vi "Diconnect.vi"(4 "error in (no error)":errorcluster, 7 "VISA resource name":refnum<visa-resource-name>) -> ()   [LabVIEW 2015]
doc: "Funcitonally the opposite of the connect block. Use this to end communication with the ESP301. This is necessary but I am not sure why."
uses:
  <userlib>/Newport ESP301/Newport ESP301.lvlib
panel:
  # "This does the opposite of the Connect Block. \nNeeds to be run at the end of any program\nwhere  you have been communicating with \nthe ESP301 box."
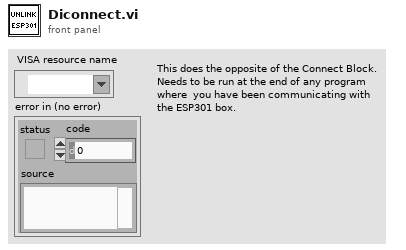
[diagram p1: front panel]
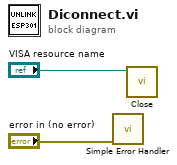
[diagram p0: block diagram]
diagram:
  n1 = call <vilib>:"Simple Error Handler.vi"("error in (no error)"="error in (no error)") -> ()  [unwired: 1 in, 8 out]
  n2 = call <userlib>:"Close.vi"("VISA resource name"="VISA resource name") -> ()  [unwired: 10 in, 1 out]
